vi "Change All Descriptionss.vi"(6 "Prompt?":bool, 9 "new":string, 10 "Path":path, 11 "VI Data in":T1[](array[typedef])) -> (1 "Changed indices":i32[](array[numeric]), 2 "adjust all":bool, 3 "VI Data out":T1[](array[typedef]))   [LabVIEW 2023, in "VI Properties Editor.lvlib"]
uses:
  VI Properties Editor.lvlib
  Cluster Data.ctl
  <vilib>/picture/picture.llb/imagedata.ctl
panel:
  # "Connector Pane"
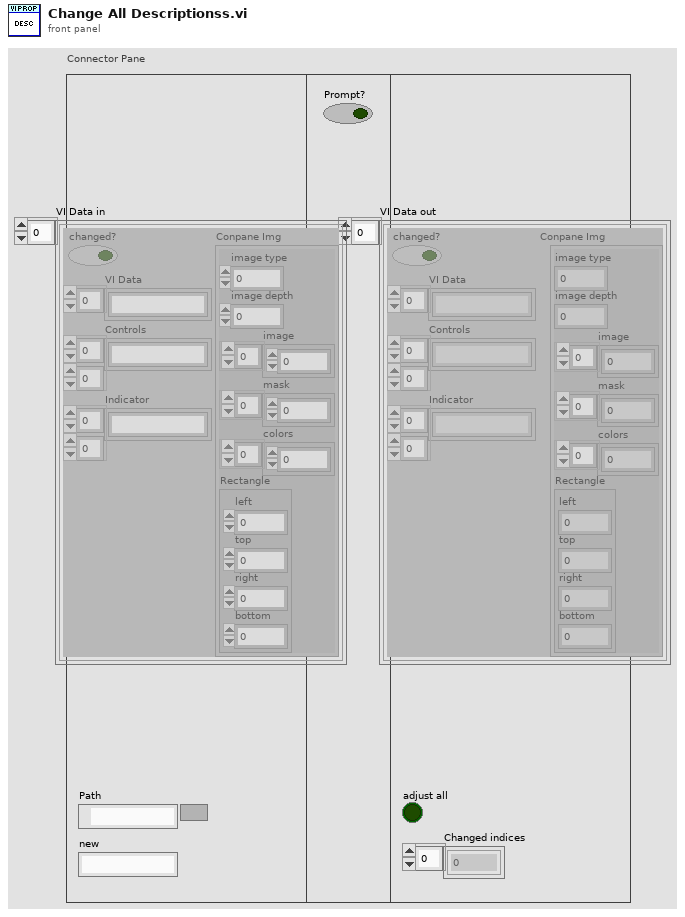
[diagram p1: front panel]
types:
  T1 = typedef "VI Properties Editor.lvlib/Cluster Data.ctl" = cluster{"changed?":bool, "VI Data":string[], "Controls":string[][], "Indicator":string[][], "Conpane Img":T2}
  T2 = typedef "imagedata.ctl" = cluster{"image type":i32, "image depth":i32, "image":u8[], "mask":u8[], "colors":u32[], "Rectangle":cluster{"left":i16, "top":i16, "right":i16, "bottom":i16}}
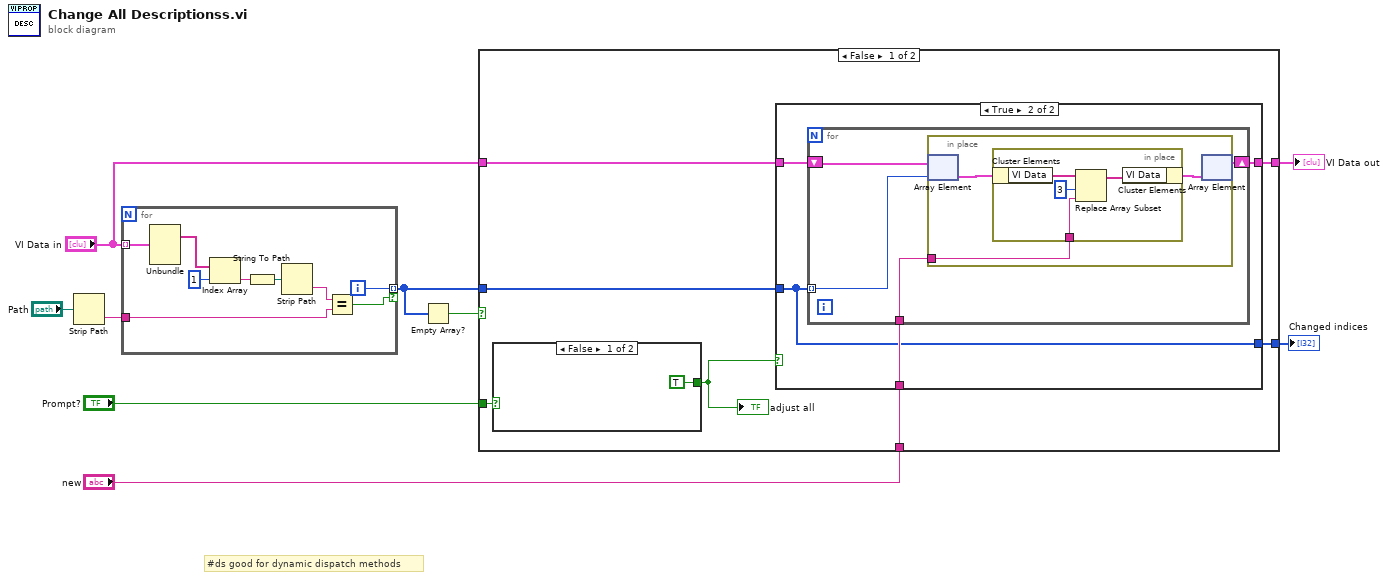
[diagram p0: block diagram]
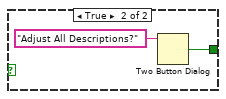
[diagram p3: hidden frame]
diagram:
  # "#ds good for dynamic dispatch methods"
  n1 = Strip Path(path="Path") -> (name=w8:string)  [unwired: 1 out]
  n2 = for {
    tunnel: "VI Data in" -> [w13] mode=indexing
    tunnel: w8 -> [w15]
    tunnel: [w12] -> w4 mode=indexing if=w11
    i -> [w12]
    n3 = Unbundle(w13) -> ("VI Data"=w10:string[])  [unwired: 4 out]
    n4 = Index Array(array=w10, index=1) -> (element=w17:string)
    n5 = String To Path(string=w17) -> (path=w16:path)
    n6 = Strip Path(path=w16) -> (name=w14:string)  [unwired: 1 out]
    n7 = Equal?(x=w14, y=w15) -> (x = y?=w11:bool)
  }
  n8 = Empty Array?(array=w4) -> (empty?=w6:bool)
  n9 = case shown="False" w6 {
    tunnel: "VI Data in" -> [w24 w45]
    tunnel: [w23 w45] -> w5
    tunnel: w4 -> [w25 _]
    tunnel: "Prompt?" -> [w22 _]
    tunnel: "new" -> [w20 _]
    tunnel: [w19 _] -> w1
    frame False {
      n10 = case shown="False" w22 {
        tunnel: [TRUE ("T button?") w43] -> w21
        frame False {
        }
        frame True {
          n11 = Two Button Dialog(message="Adjust All Descriptions?") -> (T button?=w43:bool)  [unwired: 2 in]
        }
      }
      "adjust all" <- w21
      n12 = case shown="True" w21 {
        tunnel: w25 -> [_ w27]
        tunnel: w24 -> [w26 w30]
        tunnel: [w26 w29] -> w23
        tunnel: w20 -> [_ w28]
        tunnel: [_ w27] -> w19
        frame False {
        }
        frame True {
          n13 = for {
            tunnel: w27 -> [w34] mode=indexing
            shift-right: [w33] -> w29
            shift-left: w30 -> [w31]
            tunnel: w28 -> [w32]
            n14 = in-place {
              in-place-border: w32 -> [w35]
              n15 = in-place-array #1(w31, w34) -> (w37:T1)
              n16 = in-place {
                in-place-border: w35 -> [w38]
                n17 = in-place-cluster #2(w37) -> ("VI Data"=w41:string[])
                n18 = Replace Array Subset(array=w41, new element=w38, index=3) -> (w40:string[])
                n19 = in-place-cluster #2("VI Data"=w40) -> (w36:T1)
              }
              n20 = in-place-array #1(w36) -> (w33:T1[])  [unwired: 1 out]
            }
          }
        }
      }
    }
    frame True {
    }
  }
  "VI Data out" <- w5
  "Changed indices" <- w1
